vi "Initialize.vi"(8 "error in (no error)":errorcluster, 10 "Variant/initial value":variant, 11 "SEQ name":string) -> (0 "error out":errorcluster, 3 "Ref out":refnum<queue>)   [LabVIEW 2016, in "SEQ.lvlib"]
doc: "Initialize a Single Element Queued (SEQ) based variable in variant format. Specify a <b>SEQ name</b> as identity to this variable."
uses:
  SEQ.lvlib
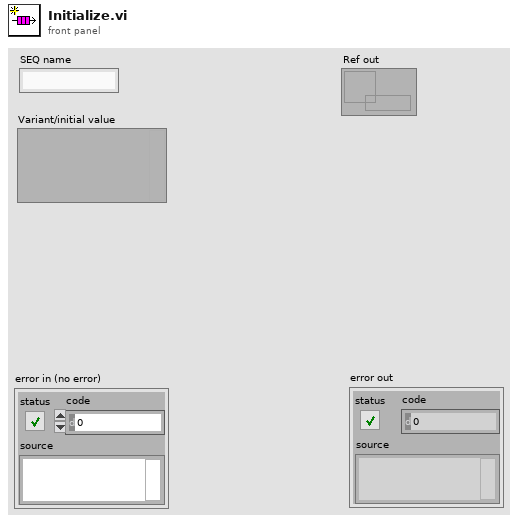
[diagram p1: front panel]
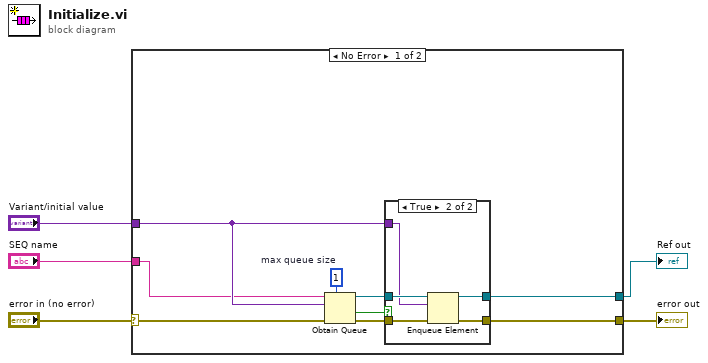
[diagram p0: block diagram]
diagram:
  n1 = case shown="No Error" "error in (no error)" {
    selector: "error in (no error)" -> [w12 w22]
    tunnel: [w10 w22] -> w5
    tunnel: "SEQ name" -> [w7 _]
    tunnel: [w9 _] -> w2
    tunnel: "Variant/initial value" -> [w8 _]
    frame No Error {
      w14 = 1  # max queue size
      n2 = Obtain Queue(max queue size (-1, unlimited)=w14, name (unnamed)=w7, element data type=w8, error in (no error)=w12) -> (queue out=w13:refnum<queue>, created new?=w6:bool, error out=w11:errorcluster)  [unwired: 1 in]
      n3 = case shown="True" w6 {
        tunnel: w13 -> [w16 w21]
        tunnel: w11 -> [w15 w20]
        tunnel: [w15 w19] -> w10
        tunnel: [w16 w18] -> w9
        tunnel: w8 -> [_ w17]
        frame False {
        }
        frame True {
          n4 = Enqueue Element(queue=w21, element=w17, error in (no error)=w20) -> (queue out=w18:refnum<queue>, error out=w19:errorcluster)  [unwired: 1 in, 1 out]
        }
      }
    }
    frame Error {
    }
  }
  "error out" <- w5
  "Ref out" <- w2
